vi "configureHWError.vi"(8 "error in (no error)":errorcluster, 11 "AtomChipHWC in":refnum<class "AtomChipHWC.lvclass">) -> (0 "error out":errorcluster, 2 "error":bool, 3 "AtomChipHWC out":refnum<class "AtomChipHWC.lvclass">)   [LabVIEW 2011, in "Hardware.lvlib" / "HWControllers.lvlib" / "AtomChipHWC.lvclass"]
uses:
  AtomChipHWC.lvclass
  AtomChipHWC.lvclass/AtomChipHWC.ctl
  Channels/Digital/DigitalOutput.lvclass
  Channels/VoltOutput/AnalogOutput.lvclass
  Channels/DDSOutput/Generic/DDSOutput.lvclass
  HWController.lvclass
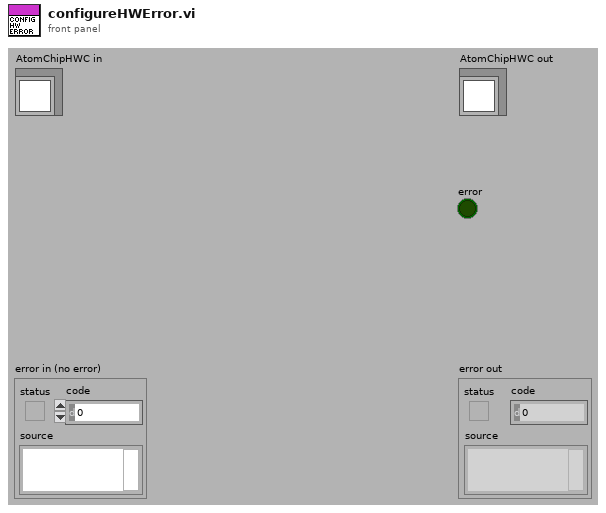
[diagram p1: front panel]
types:
  T1 = enum16{"Ready", "Compiling", "Configured", "Running", "Stopping", "Unresolved Error"}
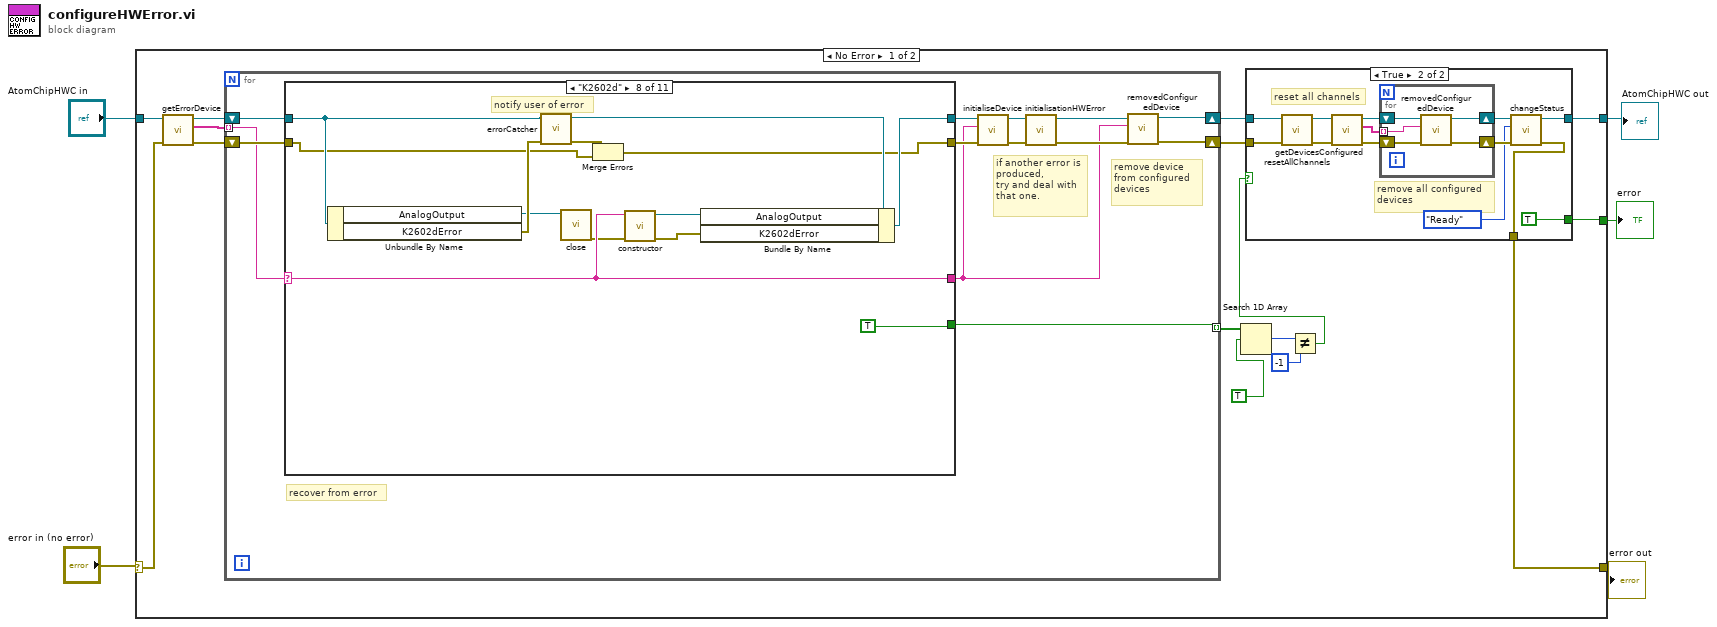
[diagram p0: block diagram]
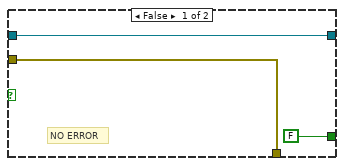
[diagram p2: hidden frame]
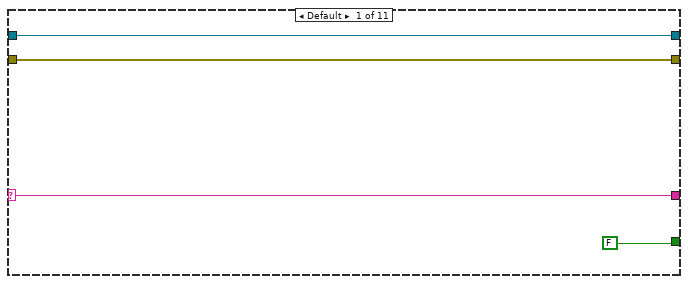
[diagram p3: hidden frame]
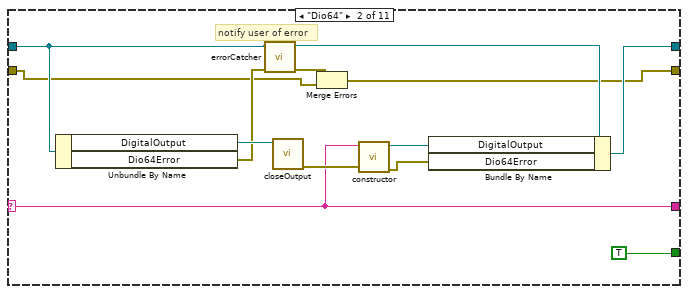
[diagram p4: hidden frame]
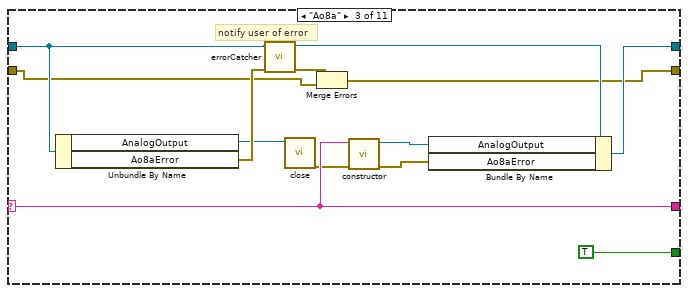
[diagram p5: hidden frame]
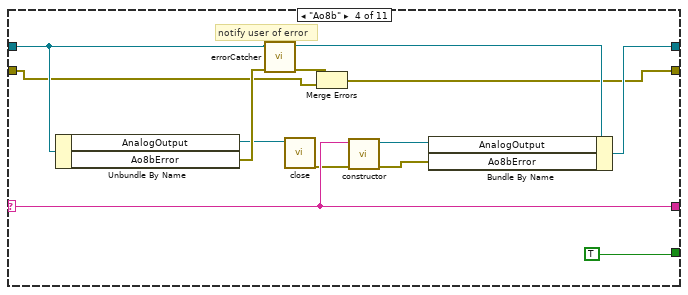
[diagram p6: hidden frame]
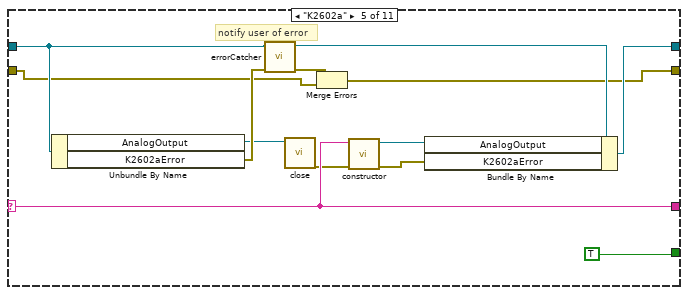
[diagram p7: hidden frame]
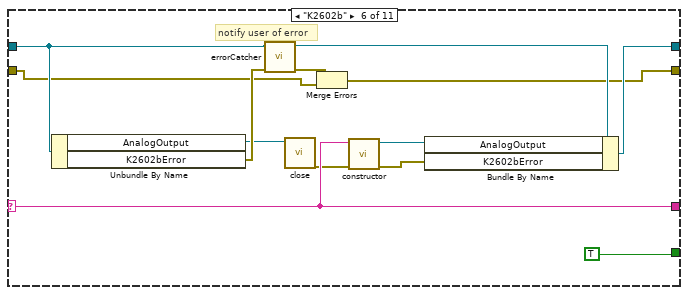
[diagram p8: hidden frame]
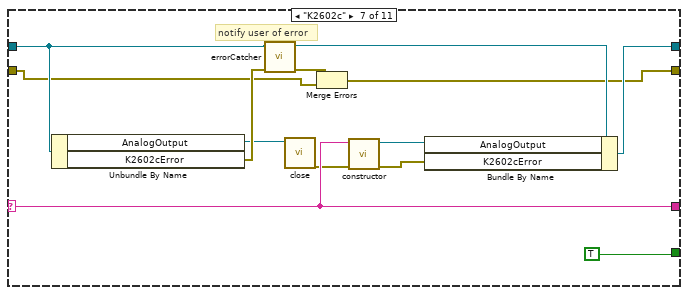
[diagram p9: hidden frame]
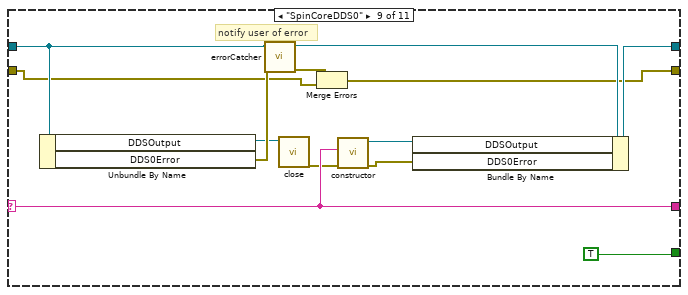
[diagram p10: hidden frame]
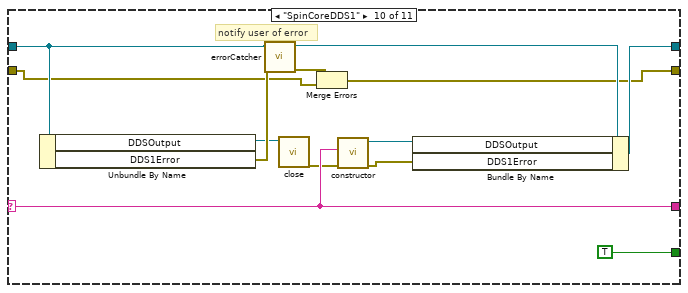
[diagram p11: hidden frame]
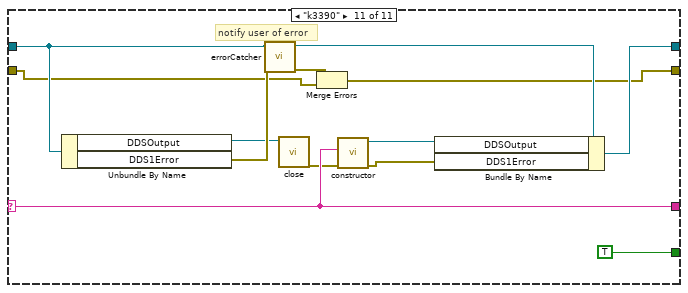
[diagram p12: hidden frame]
diagram:
  n1 = case shown="No Error" "error in (no error)" {
    selector: "error in (no error)" -> [w19 w189]
    tunnel: "AtomChipHWC in" -> [w20 w190]
    tunnel: [w12 w190] -> w3
    tunnel: [w13 w189] -> w2
    tunnel: [w11 _] -> w1
    frame No Error {
      n2 = call "getErrorDevice.vi"("error in (no error)"=w19, "AtomChipHWC in"=w20) -> ("error out"=w16:errorcluster, "Devices"=w17:string[], "AtomChipHWC out"=w18:refnum<class "AtomChipHWC.lvclass">)  [unwired: 7 in]
      n3 = for {
        tunnel: w17 -> [w52] mode=indexing
        shift-right: [w46] -> w15
        shift-left: w18 -> [w54]
        shift-right: [w45] -> w14
        shift-left: w16 -> [w53]
        tunnel: [w42] -> w10 mode=indexing
        # "remove device\nfrom configured\ndevices"
        # "if another error is\nproduced,\ntry and deal with\nthat one."
        # "recover from error"
        n4 = case shown="\"K2602d\"" w52 {
          selector: w52 -> [w56 w60 w76 w89 w102 w115 w128 w141 w152 w165 w178]
          tunnel: w54 -> [w58 w67 w84 w97 w110 w123 w136 w149 w162 w175 w188]
          tunnel: [w58 w62 w79 w92 w105 w118 w131 w144 w157 w170 w183] -> w47
          tunnel: [w57 w61 w78 w91 w104 w117 w130 w143 w156 w169 w182] -> w44
          tunnel: w53 -> [w57 w63 w80 w93 w106 w119 w132 w145 w158 w171 w184]
          tunnel: [w56 w60 w76 w89 w102 w115 w128 w141 w152 w165 w178] -> w43
          tunnel: [FALSE TRUE TRUE TRUE TRUE TRUE TRUE TRUE TRUE TRUE TRUE] -> w42
          frame Default {
          }
          frame "Dio64" {
            # "notify user of error"
            n5 = Unbundle By Name(w67) -> ("DigitalOutput"=w71:refnum<class "DigitalOutput.lvclass">, "Dio64Error"=w65:errorcluster)
            n6 = call-dynamic "errorCatcher.vi"("error in (no error)"=w65, "HWController in"=w67) -> ("error out"=w64:errorcluster, "HWController out"=w66:refnum<class "AtomChipHWC.lvclass">)  [unwired: 8 in]
            n7 = call-dynamic "closeOutput.vi"("DigitalOutput in"=w71) -> ("error out"=w70:errorcluster)  [unwired: 10 in]
            n8 = Merge Errors(w64, w63) -> (w61:errorcluster)
            n9 = call "constructor.vi"("error in (no error)"=w70, "deviceName"=w60) -> ("error out"=w68:errorcluster, "DigitalOutput out"=w69:refnum<class "DigitalOutput.lvclass">)  [unwired: 8 in]
            n10 = Bundle By Name(cluster=w66, "DigitalOutput"=w69, "Dio64Error"=w68) -> (w62:refnum<class "AtomChipHWC.lvclass">)
          }
          frame "Ao8a" {
            # "notify user of error"
            n11 = Unbundle By Name(w84) -> ("AnalogOutput"=w77:refnum<class "AnalogOutput.lvclass">, "Ao8aError"=w82:errorcluster)
            n12 = call-dynamic "errorCatcher.vi"("error in (no error)"=w82, "HWController in"=w84) -> ("error out"=w81:errorcluster, "HWController out"=w83:refnum<class "AtomChipHWC.lvclass">)  [unwired: 8 in]
            n13 = call-dynamic "close.vi"("AnalogOutput in"=w77) -> ("error out"=w75:errorcluster)  [unwired: 10 in]
            n14 = Merge Errors(w81, w80) -> (w78:errorcluster)
            n15 = call "constructor.vi"("error in (no error)"=w75, "deviceName"=w76) -> ("error out"=w73:errorcluster, "AnalogOutput out"=w74:refnum<class "AnalogOutput.lvclass">)  [unwired: 8 in]
            n16 = Bundle By Name(cluster=w83, "AnalogOutput"=w74, "Ao8aError"=w73) -> (w79:refnum<class "AtomChipHWC.lvclass">)
          }
          frame "Ao8b" {
            # "notify user of error"
            n17 = Unbundle By Name(w97) -> ("AnalogOutput"=w90:refnum<class "AnalogOutput.lvclass">, "Ao8bError"=w95:errorcluster)
            n18 = call-dynamic "errorCatcher.vi"("error in (no error)"=w95, "HWController in"=w97) -> ("error out"=w94:errorcluster, "HWController out"=w96:refnum<class "AtomChipHWC.lvclass">)  [unwired: 8 in]
            n19 = call-dynamic "close.vi"("AnalogOutput in"=w90) -> ("error out"=w88:errorcluster)  [unwired: 10 in]
            n20 = Merge Errors(w94, w93) -> (w91:errorcluster)
            n21 = call "constructor.vi"("error in (no error)"=w88, "deviceName"=w89) -> ("error out"=w86:errorcluster, "AnalogOutput out"=w87:refnum<class "AnalogOutput.lvclass">)  [unwired: 8 in]
            n22 = Bundle By Name(cluster=w96, "AnalogOutput"=w87, "Ao8bError"=w86) -> (w92:refnum<class "AtomChipHWC.lvclass">)
          }
          frame "K2602a" {
            # "notify user of error"
            n23 = Unbundle By Name(w110) -> ("AnalogOutput"=w103:refnum<class "AnalogOutput.lvclass">, "K2602aError"=w108:errorcluster)
            n24 = call-dynamic "errorCatcher.vi"("error in (no error)"=w108, "HWController in"=w110) -> ("error out"=w107:errorcluster, "HWController out"=w109:refnum<class "AtomChipHWC.lvclass">)  [unwired: 8 in]
            n25 = call-dynamic "close.vi"("AnalogOutput in"=w103) -> ("error out"=w101:errorcluster)  [unwired: 10 in]
            n26 = Merge Errors(w107, w106) -> (w104:errorcluster)
            n27 = call "constructor.vi"("error in (no error)"=w101, "deviceName"=w102) -> ("error out"=w99:errorcluster, "AnalogOutput out"=w100:refnum<class "AnalogOutput.lvclass">)  [unwired: 8 in]
            n28 = Bundle By Name(cluster=w109, "AnalogOutput"=w100, "K2602aError"=w99) -> (w105:refnum<class "AtomChipHWC.lvclass">)
          }
          frame "K2602b" {
            # "notify user of error"
            n29 = Unbundle By Name(w123) -> ("AnalogOutput"=w116:refnum<class "AnalogOutput.lvclass">, "K2602bError"=w121:errorcluster)
            n30 = call-dynamic "errorCatcher.vi"("error in (no error)"=w121, "HWController in"=w123) -> ("error out"=w120:errorcluster, "HWController out"=w122:refnum<class "AtomChipHWC.lvclass">)  [unwired: 8 in]
            n31 = call-dynamic "close.vi"("AnalogOutput in"=w116) -> ("error out"=w114:errorcluster)  [unwired: 10 in]
            n32 = Merge Errors(w120, w119) -> (w117:errorcluster)
            n33 = call "constructor.vi"("error in (no error)"=w114, "deviceName"=w115) -> ("error out"=w112:errorcluster, "AnalogOutput out"=w113:refnum<class "AnalogOutput.lvclass">)  [unwired: 8 in]
            n34 = Bundle By Name(cluster=w122, "AnalogOutput"=w113, "K2602bError"=w112) -> (w118:refnum<class "AtomChipHWC.lvclass">)
          }
          frame "K2602c" {
            # "notify user of error"
            n35 = Unbundle By Name(w136) -> ("AnalogOutput"=w129:refnum<class "AnalogOutput.lvclass">, "K2602cError"=w134:errorcluster)
            n36 = call-dynamic "errorCatcher.vi"("error in (no error)"=w134, "HWController in"=w136) -> ("error out"=w133:errorcluster, "HWController out"=w135:refnum<class "AtomChipHWC.lvclass">)  [unwired: 8 in]
            n37 = call-dynamic "close.vi"("AnalogOutput in"=w129) -> ("error out"=w127:errorcluster)  [unwired: 10 in]
            n38 = Merge Errors(w133, w132) -> (w130:errorcluster)
            n39 = call "constructor.vi"("error in (no error)"=w127, "deviceName"=w128) -> ("error out"=w125:errorcluster, "AnalogOutput out"=w126:refnum<class "AnalogOutput.lvclass">)  [unwired: 8 in]
            n40 = Bundle By Name(cluster=w135, "AnalogOutput"=w126, "K2602cError"=w125) -> (w131:refnum<class "AtomChipHWC.lvclass">)
          }
          frame "K2602d" {
            # "notify user of error"
            n41 = Unbundle By Name(w149) -> ("AnalogOutput"=w142:refnum<class "AnalogOutput.lvclass">, "K2602dError"=w147:errorcluster)
            n42 = call-dynamic "errorCatcher.vi"("error in (no error)"=w147, "HWController in"=w149) -> ("error out"=w146:errorcluster, "HWController out"=w148:refnum<class "AtomChipHWC.lvclass">)  [unwired: 8 in]
            n43 = call-dynamic "close.vi"("AnalogOutput in"=w142) -> ("error out"=w140:errorcluster)  [unwired: 10 in]
            n44 = Merge Errors(w146, w145) -> (w143:errorcluster)
            n45 = call "constructor.vi"("error in (no error)"=w140, "deviceName"=w141) -> ("error out"=w138:errorcluster, "AnalogOutput out"=w139:refnum<class "AnalogOutput.lvclass">)  [unwired: 8 in]
            n46 = Bundle By Name(cluster=w148, "AnalogOutput"=w139, "K2602dError"=w138) -> (w144:refnum<class "AtomChipHWC.lvclass">)
          }
          frame "SpinCoreDDS0" {
            # "notify user of error"
            n47 = Unbundle By Name(w162) -> ("DDSOutput"=w155:refnum<class "DDSOutput.lvclass">, "DDS0Error"=w160:errorcluster)
            n48 = call-dynamic "errorCatcher.vi"("error in (no error)"=w160, "HWController in"=w162) -> ("error out"=w159:errorcluster, "HWController out"=w161:refnum<class "AtomChipHWC.lvclass">)  [unwired: 8 in]
            n49 = call-dynamic "close.vi"("DDSOutput in"=w155) -> ("error out"=w151:errorcluster)  [unwired: 10 in]
            n50 = Merge Errors(w159, w158) -> (w156:errorcluster)
            n51 = call "constructor.vi"("error in (no error)"=w151, "device"=w152) -> ("error out"=w153:errorcluster, "DDSOutput out"=w154:refnum<class "DDSOutput.lvclass">)  [unwired: 8 in]
            n52 = Bundle By Name(cluster=w161, "DDSOutput"=w154, "DDS0Error"=w153) -> (w157:refnum<class "AtomChipHWC.lvclass">)
          }
          frame "SpinCoreDDS1" {
            # "notify user of error"
            n53 = Unbundle By Name(w175) -> ("DDSOutput"=w168:refnum<class "DDSOutput.lvclass">, "DDS1Error"=w173:errorcluster)
            n54 = call-dynamic "errorCatcher.vi"("error in (no error)"=w173, "HWController in"=w175) -> ("error out"=w172:errorcluster, "HWController out"=w174:refnum<class "AtomChipHWC.lvclass">)  [unwired: 8 in]
            n55 = call-dynamic "close.vi"("DDSOutput in"=w168) -> ("error out"=w164:errorcluster)  [unwired: 10 in]
            n56 = Merge Errors(w172, w171) -> (w169:errorcluster)
            n57 = call "constructor.vi"("error in (no error)"=w164, "device"=w165) -> ("error out"=w166:errorcluster, "DDSOutput out"=w167:refnum<class "DDSOutput.lvclass">)  [unwired: 8 in]
            n58 = Bundle By Name(cluster=w174, "DDSOutput"=w167, "DDS1Error"=w166) -> (w170:refnum<class "AtomChipHWC.lvclass">)
          }
          frame "k3390" {
            # "notify user of error"
            n59 = Unbundle By Name(w188) -> ("DDSOutput"=w181:refnum<class "DDSOutput.lvclass">, "DDS1Error"=w186:errorcluster)
            n60 = call-dynamic "errorCatcher.vi"("error in (no error)"=w186, "HWController in"=w188) -> ("error out"=w185:errorcluster, "HWController out"=w187:refnum<class "AtomChipHWC.lvclass">)  [unwired: 8 in]
            n61 = call-dynamic "close.vi"("DDSOutput in"=w181) -> ("error out"=w177:errorcluster)  [unwired: 10 in]
            n62 = Merge Errors(w185, w184) -> (w182:errorcluster)
            n63 = call "constructor.vi"("error in (no error)"=w177, "device"=w178) -> ("error out"=w179:errorcluster, "DDSOutput out"=w180:refnum<class "DDSOutput.lvclass">)  [unwired: 8 in]
            n64 = Bundle By Name(cluster=w187, "DDSOutput"=w180, "DDS1Error"=w179) -> (w183:refnum<class "AtomChipHWC.lvclass">)
          }
        }
        n65 = call "initialiseDevice.vi"("error in (no error)"=w44, "deviceName"=w43, "AtomChipHWC in"=w47) -> ("error out"=w50:errorcluster, "AtomChipHWC out"=w51:refnum<class "AtomChipHWC.lvclass">)  [unwired: 7 in]
        n66 = call-dynamic "initialisationHWError.vi"("error in (no error)"=w50, "AtomChipHWC in"=w51) -> ("error out"=w48:errorcluster, "AtomChipHWC out"=w49:refnum<class "AtomChipHWC.lvclass">)  [unwired: 8 in]
        n67 = call-dynamic "removedConfiguredDevice.vi"("error in (no error)"=w48, "device"=w43, "HWController in"=w49) -> ("error out"=w45:errorcluster, "HWController out"=w46:refnum<class "AtomChipHWC.lvclass">)  [unwired: 7 in]
      }
      n68 = Search 1D Array(1D array=w10, element=TRUE) -> (index of element=w8:i32)  [unwired: 1 in]
      n69 = Not Equal?(x=w8, y=-1) -> (x != y?=w6:bool)
      n70 = case shown="True" w6 {
        tunnel: w15 -> [w23 w36]
        tunnel: w14 -> [w22 w35]
        tunnel: [w22 w25] -> w13
        tunnel: [w23 w27] -> w12
        tunnel: [FALSE TRUE] -> w11
        frame False {
          # "NO ERROR"
        }
        frame True {
          # "remove all configured\ndevices"
          # "reset all channels"
          n71 = call-dynamic "resetAllChannels.vi"("error in (no error)"=w35, "AtomChipHWC in"=w36) -> ("error out"=w33:errorcluster, "AtomChipHWC out"=w34:refnum<class "AtomChipHWC.lvclass">)  [unwired: 8 in]
          n72 = call "getDevicesConfigured.vi"("error in (no error)"=w33, "HWController.lvclass in"=w34) -> ("error out"=w31:errorcluster, "devicesConfigured"=w30:string[], "HWController.lvclass out"=w32:refnum<class "AtomChipHWC.lvclass">)  [unwired: 7 in]
          n73 = for {
            shift-right: [w40] -> w28
            shift-left: w32 -> [w41]
            shift-right: [w38] -> w26
            shift-left: w31 -> [w39]
            tunnel: w30 -> [w37] mode=indexing
            n74 = call-dynamic "removedConfiguredDevice.vi"("error in (no error)"=w39, "device"=w37, "HWController in"=w41) -> ("error out"=w38:errorcluster, "HWController out"=w40:refnum<class "AtomChipHWC.lvclass">)  [unwired: 7 in]
          }
          n75 = call "changeStatus.vi"("error in (no error)"=w26, "status"=T1."Ready", "HWController in"=w28) -> ("error out"=w25:errorcluster, "HWController out"=w27:refnum<class "AtomChipHWC.lvclass">)  [unwired: 7 in]
        }
      }
    }
    frame Error {
    }
  }
  "error out" <- w2
  "AtomChipHWC out" <- w3
  "error" <- w1
